vi "XYZStage-Set max speed command.vi"(8 "Error In":errorcluster, 9 "XYZ Stage data":T2={"Command"=enum."Initialize", "Channel"="Z", "X"=0.0, "Y"=0.0, "Z"=0.0, "Speed"=0, "Zero"=FALSE, "Use acknowledgement?"=TRUE} {"Speed" format="Speed= %.0f"; "Z" format="Z= %#_g"; "Y" format="Y= %#_g"; "X" format="X= %#_g"}, 10 "Z Stage":T1, 11 "XYZ Stage config":T5={"COM port"="COM7", "Baudrate"=0, "Type"=""}) -> (0 "Error Out":errorcluster)   [LabVIEW 2020]
uses:
  Typedefs/XY Stage config cluster.ctl
  Typedefs/XYZ stage data.ctl
  Typedefs/XYZ stage states.ctl
  Typedefs/XYZ channel ring.ctl
  Typedefs/Z Stage config cluster.ctl
  Global Variables/General Globals.vi
panel:
  out "read string":string
  out "Set max speed command string":string
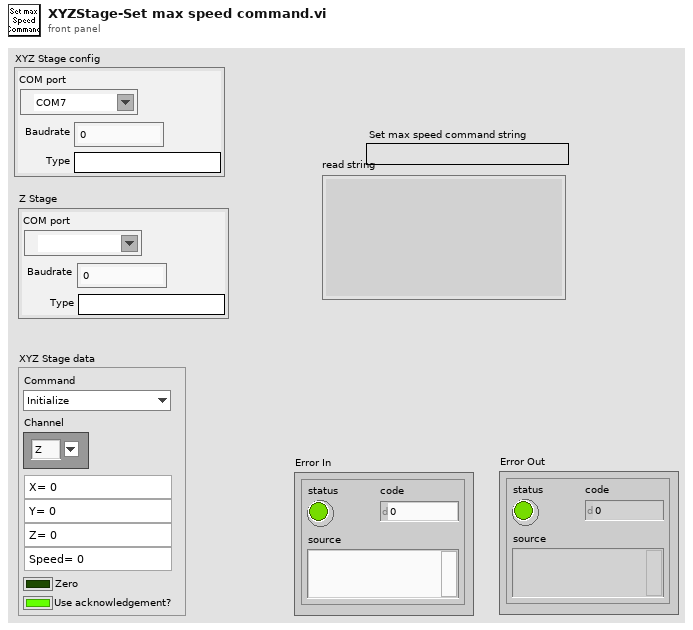
[diagram p1: front panel]
types:
  T1 = typedef "Z Stage config cluster.ctl" = cluster{"COM port":refnum<visa-resource-name>, "Baudrate":i32, "Type":string}
  T2 = typedef "XYZ stage data.ctl" = cluster{"Command":T3, "Channel":T4, "X":sgl, "Y":sgl, "Z":sgl, "Speed":i32, "Zero":bool, "Use acknowledgement?":bool}
  T3 = typedef "XYZ stage states.ctl" = enum16{"Dequeue", "Initialize", "Read Position", "Read Speed Setting", "Move", "Set Max Speed", "Reset Axis", "Stop all movement"}
  T4 = typedef "XYZ channel ring.ctl" = string
  T5 = typedef "XY Stage config cluster.ctl" = cluster{"COM port":refnum<visa-resource-name>, "Baudrate":i32, "Type":string}
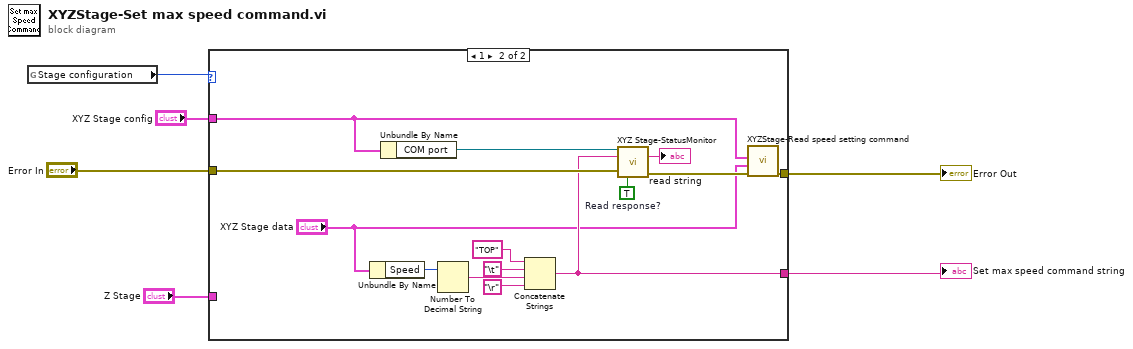
[diagram p0: block diagram]
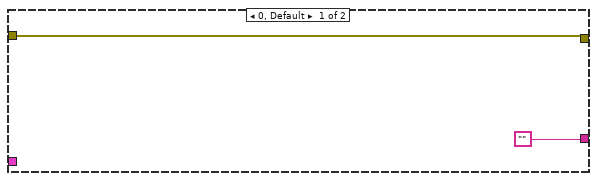
[diagram p2: hidden frame]
diagram:
  n1 = global read "General Globals.vi" "Stage configuration"() -> (w2:i32)
  n2 = case shown="1" w2 {
    tunnel: "Error In" -> [w7 w22]
    tunnel: ["" w14] -> w5
    tunnel: [w7 w12] -> w4
    tunnel: "XYZ Stage config" -> [_ w9]
    tunnel: "Z Stage" -> [_ _]
    frame 0, Default {
    }
    frame 1 {
      w21 = TRUE  # Read response?
      n3 = Unbundle By Name("XYZ Stage data") -> ("Speed"=w16:i32)
      n4 = Unbundle By Name(w9) -> ("COM port"=w15:refnum<visa-resource-name>)
      n5 = Number To Decimal String(number=w16) -> (decimal integer string=w20:string)  [unwired: 1 in]
      n6 = Concatenate Strings("TOP" ("decimal integer string"), "\t" ("Tab Constant"), w20, "\r" ("Carriage Return Constant")) -> (w14:string)
      n7 = call "XYZ Stage-StatusMonitor.vi"("VISA resource name"=w15, "string to write"=w14, "Error In"=w22, "Read response? (T)"=w21) -> ("read string"=→"read string":string, "Error Out"=w13:errorcluster)  [unwired: 7 in, 3 out]
      n8 = call "XYZStage-Read speed setting command.vi"("error in (no error)"=w13, "XYZ Stage data to queue"="XYZ Stage data", "Z Stage"=w9) -> ("error out"=w12:errorcluster)  [unwired: 8 in]
    }
  }
  "Error Out" <- w4
  "Set max speed command string" <- w5
